vi "Generate Axis and Circle.vi"(1 "Blank picture":picture) -> (0 "Output picture":picture)   [LabVIEW 2014]
panel:
  in  "color(black)":u32(colorbox)=7171459
  in  "desired font(Application) 4":T1(ring)
  in  "[user-specified font] 4":T2={"Font Name:"="Application Font", "Size"=30, "Strikeout?"=FALSE, "Italic?"=FALSE, "Underline?"=FALSE, "Outline?"=FALSE, "Shadow?"=FALSE, "Bold?"=TRUE}
  in  "origin 4":cluster{"x":i16, "y":i16}={"x"=285, "y"=90}
  in  "text 4":string="D-"
  in  "desired font(Application) 3":T1(ring)
  in  "[user-specified font] 3":T2={"Font Name:"="Application Font", "Size"=30, "Strikeout?"=FALSE, "Italic?"=FALSE, "Underline?"=FALSE, "Outline?"=FALSE, "Shadow?"=FALSE, "Bold?"=TRUE}
  in  "origin 3":cluster{"x":i16, "y":i16}={"x"=285, "y"=480}
  in  "text 3":string="D+"
  in  "desired font(Application) 2":T1(ring)
  in  "[user-specified font] 2":T2={"Font Name:"="Application Font", "Size"=30, "Strikeout?"=FALSE, "Italic?"=FALSE, "Underline?"=FALSE, "Outline?"=FALSE, "Shadow?"=FALSE, "Bold?"=TRUE}
  in  "origin 2":cluster{"x":i16, "y":i16}={"x"=95, "y"=285}
  in  "text 2":string="A-"
  in  "desired font(Application)":T1(ring)
  in  "[user-specified font]":T2={"Font Name:"="Application Font", "Size"=30, "Strikeout?"=FALSE, "Italic?"=FALSE, "Underline?"=FALSE, "Outline?"=FALSE, "Shadow?"=FALSE, "Bold?"=TRUE}
  in  "origin":cluster{"x":i16, "y":i16}={"x"=485, "y"=285}
  in  "text":string="A+"
  in  "fill?(F)":bool=TRUE
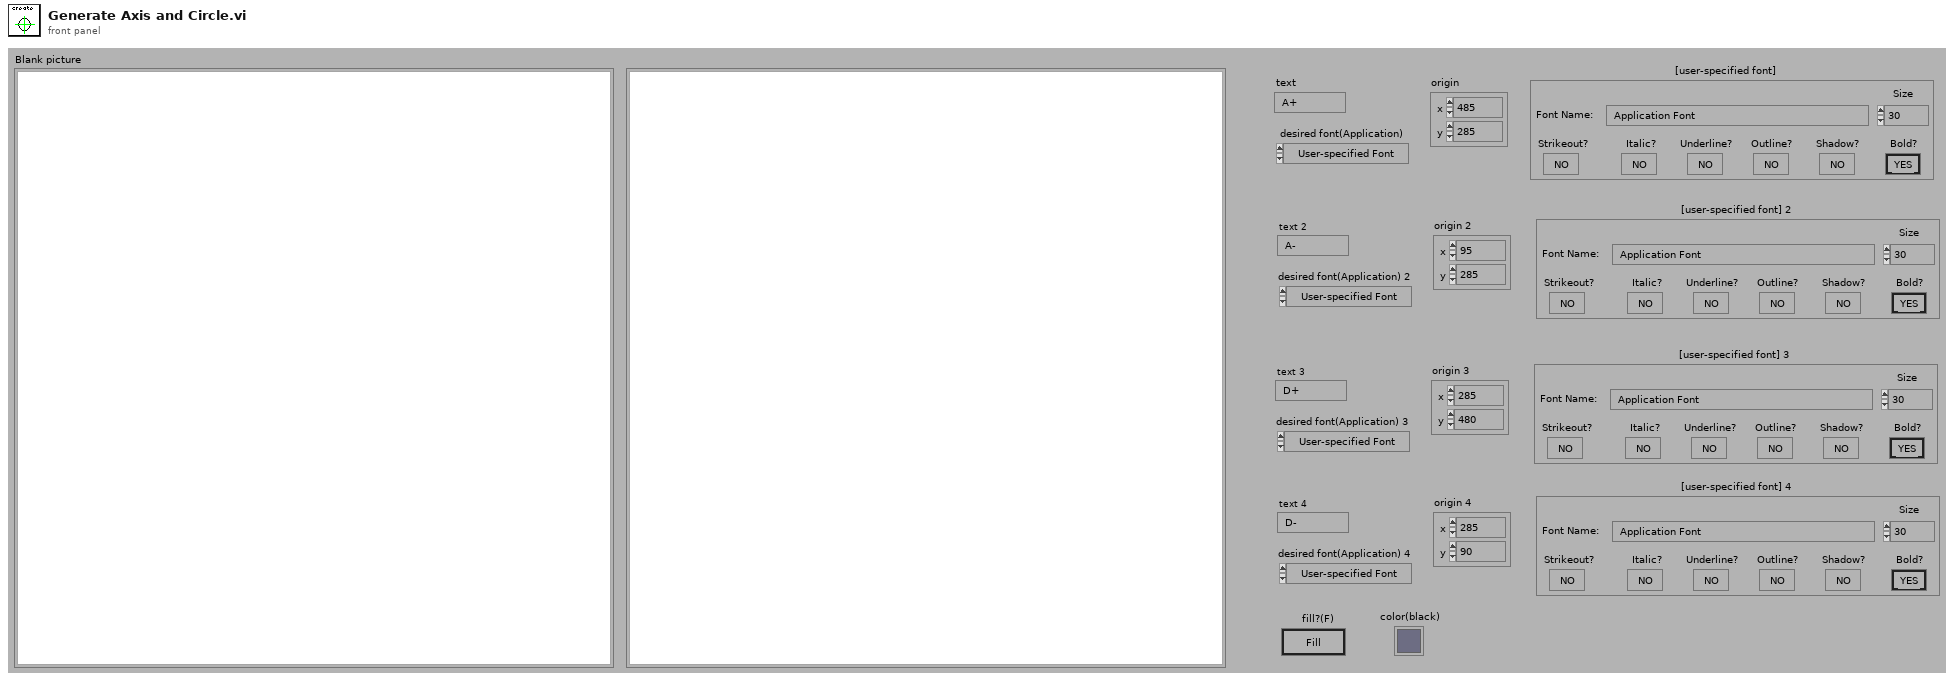
[diagram p1: front panel]
types:
  T1 = enum16{"User-specified Font", "Application Font", "System Font", "Dialog Font"}
  T2 = cluster{"Font Name:":string, "Size":i16, "Strikeout?":bool, "Italic?":bool, "Underline?":bool, "Outline?":bool, "Shadow?":bool, "Bold?":bool}
  T3 = cluster{"Width":u16, "Style":enum32{"Solid", "Dash", "Dot", "DashDot", "DashDotDot"}}
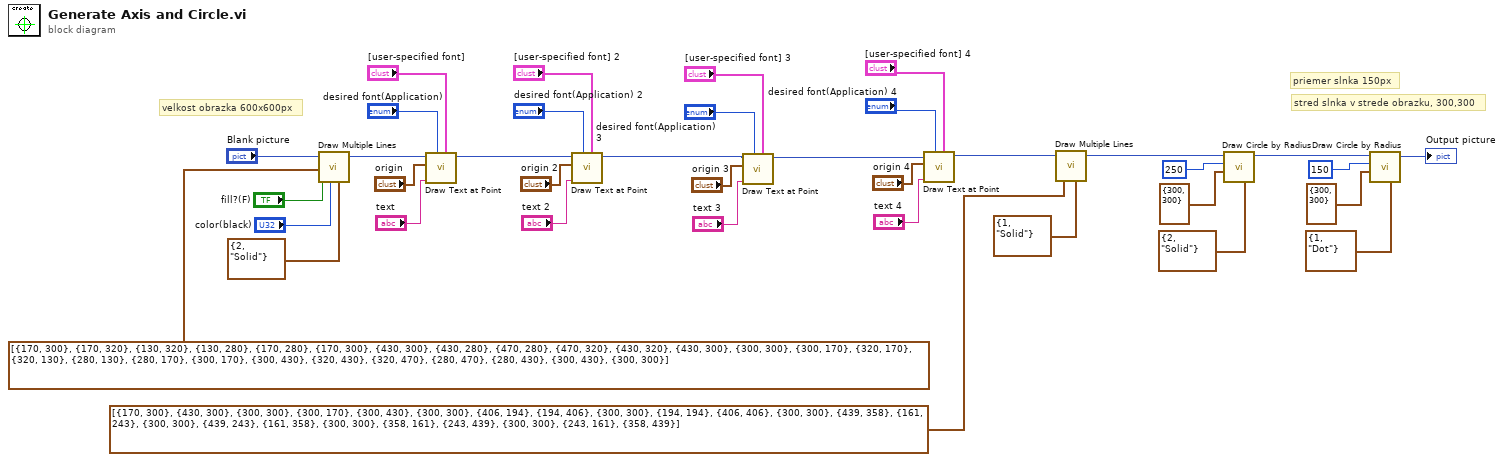
[diagram p0: block diagram]
diagram:
  # "stred slnka v strede obrazku, 300,300"
  # "priemer slnka 150px"
  # "velkost obrazka 600x600px"
  n1 = call <vilib>:"Draw Multiple Lines.vi"("picture"="Blank picture", "line endpoints"=cluster{i32, i32}[] [{170, 300}, {170, 320}, {130, 320}, {130, 280}, {170, 280}, {170, 300}, {430, 300}, {430, 280}, {470, 280}, {470, 320}, {430, 320}, {430, 300}, {300, 300}, {300, 170}, {320, 170}, {320, 130}, {280, 130}, {280, 170}, {300, 170}, {300, 430}, {320, 430}, {320, 470}, {280, 470}, {280, 430}, {300, 430}, {300, 300}], "fill?(F)"="fill?(F)", "color(black)"="color(black)", "pen"=T3 {"Width"=2, "Style"=enum."Solid"} ("pen 2")) -> ("new picture"=w25:picture)  [unwired: 4 in]
  n2 = call <vilib>:"Draw Text at Point.vi"("[user-specified font]"="[user-specified font]", "desired font(Application)"="desired font(Application)", "text"="text", "origin"="origin", "picture"=w25) -> ("new picture"=w16:picture)  [unwired: 5 in, 1 out]
  n3 = call <vilib>:"Draw Text at Point.vi"("[user-specified font]"="[user-specified font] 2", "desired font(Application)"="desired font(Application) 2", "text"="text 2", "origin"="origin 2", "picture"=w16) -> ("new picture"=w7:picture)  [unwired: 5 in, 1 out]
  n4 = call <vilib>:"Draw Text at Point.vi"("[user-specified font]"="[user-specified font] 3", "desired font(Application)"="desired font(Application) 3", "text"="text 3", "origin"="origin 3", "picture"=w7) -> ("new picture"=w6:picture)  [unwired: 5 in, 1 out]
  n5 = call <vilib>:"Draw Text at Point.vi"("[user-specified font]"="[user-specified font] 4", "desired font(Application)"="desired font(Application) 4", "text"="text 4", "origin"="origin 4", "picture"=w6) -> ("new picture"=w5:picture)  [unwired: 5 in, 1 out]
  n6 = call <vilib>:"Draw Multiple Lines.vi"("picture"=w5, "line endpoints"=cluster{i32, i32}[] [{170, 300}, {430, 300}, {300, 300}, {300, 170}, {300, 430}, {300, 300}, {406, 194}, {194, 406}, {300, 300}, {194, 194}, {406, 406}, {300, 300}, {439, 358}, {161, 243}, {300, 300}, {439, 243}, {161, 358}, {300, 300}, {358, 161}, {243, 439}, {300, 300}, {243, 161}, {358, 439}], "pen"=T3 {"Width"=1, "Style"=enum."Solid"}) -> ("new picture"=w4:picture)  [unwired: 6 in]
  n7 = call <vilib>:"Draw Circle by Radius.vi"("pen"=T3 {"Width"=2, "Style"=enum."Solid"}, "pixel center"=cluster{"vertical":i16, "horizontal":i16} {"vertical"=300, "horizontal"=300}, "radius"=i16 250, "picture"=w4) -> ("new picture"=w26:picture)  [unwired: 7 in]
  n8 = call <vilib>:"Draw Circle by Radius.vi"("pen"=T3 {"Width"=1, "Style"=enum."Dot"}, "pixel center"=cluster{"horizontal":i16, "vertical":i16} {"horizontal"=300, "vertical"=300}, "radius"=i16 150, "picture"=w26) -> ("new picture"=→"Output picture":picture)  [unwired: 7 in]
